vi "ReplaceSelfClosingStructureElements.vi"(11 "String In":string) -> (3 "String Out":string)   [LabVIEW 2018]
uses:
  <vilib>/regexp/Match Regular Expression.xnode
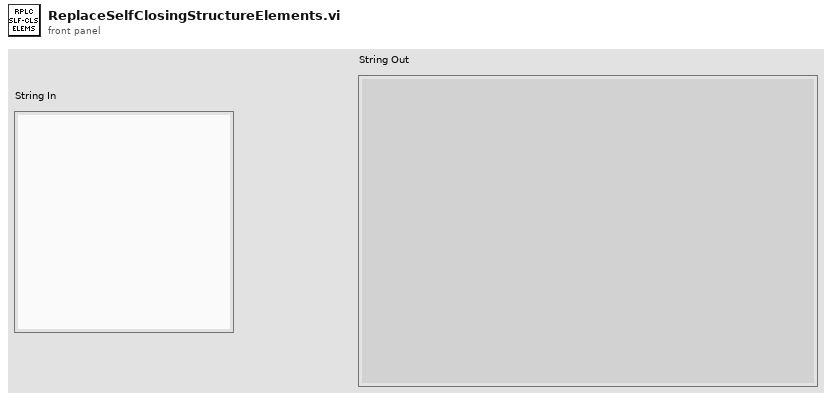
[diagram p1: front panel]
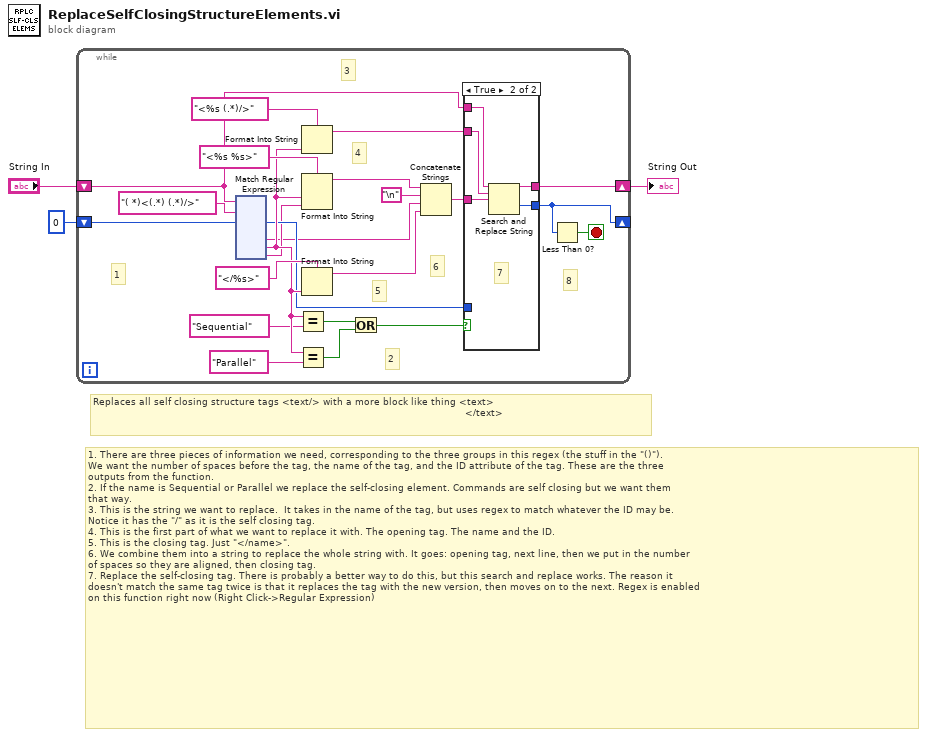
[diagram p0: block diagram]
diagram:
  # "1. There are three pieces of information we need, corresponding to the three groups in this regex (the stuff in the \"()\").\nWe want the number of spaces before the tag, the name of the tag, and the ID attribute of the tag. These are the three\noutputs from the function.\n2. If the name is Sequential or Parallel we replace the self-closing element. Commands are self closing but we want them\nthat way.\n3. This is the string we want to replace.  It takes in the name of the tag, but uses regex to match whatever the ID may be. \nNotice it has the \"/\" as it is the self closing tag.\n4. This is the first part of what we want to replace it with. The opening tag. The name and the ID. \n5. This is the closing tag. Just \"</name>\".\n6. We combine them into a string to replace the whole string with. It goes: opening tag, next line, then we put in the number\nof spaces so they are aligned, then closing tag.\n7. Replace the self-closing tag. There is probably a better way to do this, but this search and replace works. The reason it\ndoesn't match the same tag twice is that it replaces the tag with the new version, then moves on to the next. Regex is enabled\non this function right now (Right Click->Regular Expression)"
  # "Replaces all self closing structure tags <text/> with a more block like thing <text>\n                                                                                                                            </text>"
  n1 = while {
    shift-right: [w26] -> w1
    shift-left: "String In" -> [w24]
    shift-right: [w22] -> _
    shift-left: 0 -> [w23]
    stop <- w25 stop-if-true
    # "8"
    # "6"
    # "5"
    # "4"
    # "3"
    # "2"
    # "1"
    n2 = xnode "Match Regular Expression"("input string"=w24, "regular expression"="( *)<(.*) (.*)/>" ("format string"), "offset (0)"=w23) -> ("offset past match"=w6:i32, "submatch 1"=w4:string, "submatch 2"=w14:string, "submatch 3"=w5:string)  [unwired: 3 in, 4 out]
    n3 = Equal?(x=w14, y="Sequential") -> (x = y?=w11:bool)
    n4 = Equal?(x=w14, y="Parallel") -> (x = y?=w10:bool)
    n5 = Format Into String(format string="<%s (.*)/>" ("search string"), w14) -> (resulting string=w9:string)  [unwired: 2 in, 1 out]
    n6 = Format Into String(format string="<%s %s>" ("replace string (\"\")"), w14, w5) -> (resulting string=w19:string)  [unwired: 2 in, 1 out]
    n7 = Format Into String(format string="</%s>" ("replace string (\"\")"), w14) -> (resulting string=w16:string)  [unwired: 2 in, 1 out]
    n8 = Or(x=w11, y=w10) -> (x .or. y?=w7:bool)
    n9 = Concatenate Strings(w19, "\n", w4, w16) -> (w8:string)
    n10 = case shown="True" w7 {
      tunnel: [w28 w33] -> w26
      tunnel: w24 -> [w28 w32]
      tunnel: [w27 w31] -> w22
      tunnel: w9 -> [_ w30]
      tunnel: w8 -> [_ w29]
      tunnel: w6 -> [w27 _]
      frame False {
      }
      frame True {
        # "7"
        n11 = Search and Replace String(input string=w32, search string=w30, replace string=w29) -> (result string=w33:string, offset past replacement=w31:i32)  [unwired: 5 in, 2 out]
      }
    }
    n12 = Less Than 0?(x=w22) -> (x < 0?=w25:bool)
  }
  "String Out" <- w1
